vi "Lab3_5Var.vi"() -> ()   [LabVIEW 2022 SP3]
panel:
  out "String 2":string
  in  "String":string
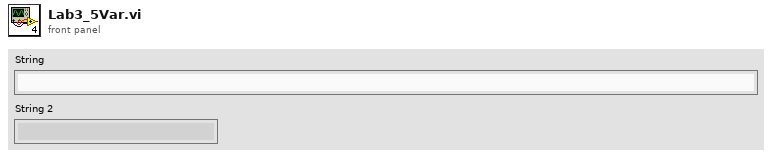
[diagram p1: front panel]
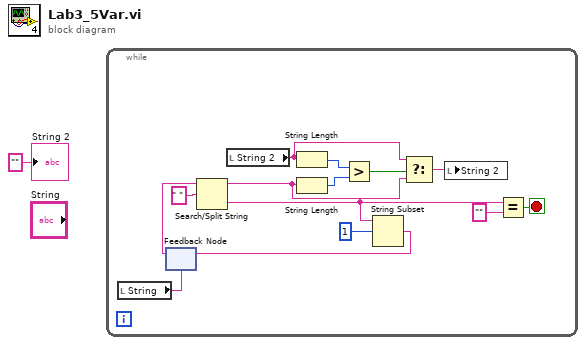
[diagram p0: block diagram]
diagram:
  n1 = while {
    stop <- w5 stop-if-true
    n2 = local read "String"() -> (w3:string)
    n3 = feedback #1(w3) -> (w14:string)
    n4 = Search/Split String(string=w14, search string/char (-)=" ") -> (substring before match=w9:string, match + rest of string=w4:string)  [unwired: 1 in, 1 out]
    n5 = local read "String 2"() -> (w10:string)
    n6 = String Length(string=w10) -> (length=w11:i32)
    n7 = String Length(string=w9) -> (length=w2:i32)
    n8 = Greater?(x=w11, y=w2) -> (0:w12:bool)
    n9 = String Subset(string=w4, offset (0)=1) -> (substring=w7:string)  [unwired: 1 in]
    n10 = feedback-in #1(w7) -> ()
    n11 = Select(t=w10, s=w12, f=w9) -> (s? t:f=w8:string)
    n12 = local write "String 2"(w8) -> ()
    n13 = Equal?(x=w4, y="") -> (x = y?=w5:bool)
  }
  "String 2" <- "" ("String 2")
